vi "GetImage.vi"(0 "XRef":T4, 1 "State In":T3={"Type"=variant(bool FALSE)}) -> (14 "Image":T2, 15 "Fatal Error Out":T1)   [LabVIEW 2017, in "WriteTag.xnode"]
doc: "Write Tag XNode script that returns the picture drawn on the node."
uses:
  WriteTag.xnode
  <vilib>/XNodeSupport/XNodeXNodeRef.ctl
  State.ctl
  <vilib>/XNodeSupport/XNodeImage.ctl
  <vilib>/XNodeSupport/XNodeErrorCluster.ctl
  <vilib>/XNodeSupport/NI_XNodeSupport.lvlib
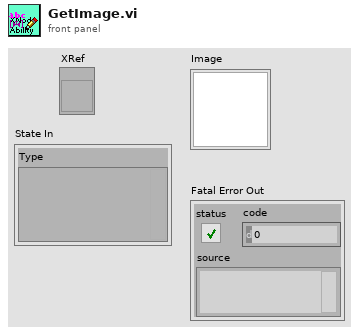
[diagram p1: front panel]
types:
  T1 = typedef "NI_XNodeSupport.lvlib/XNodeErrorCluster.ctl" = errorcluster
  T2 = typedef "NI_XNodeSupport.lvlib/XNodeImage.ctl" = picture
  T3 = typedef "WriteTag.xnode/State.ctl" = cluster{"Type":variant}
  T4 = typedef "NI_XNodeSupport.lvlib/XNodeXNodeRef.ctl" = refnum<vi>
  T5 = typedef "imagedata.ctl" = cluster{"image type":i32, "image depth":i32, "image":u8[], "mask":u8[], "colors":u32[], "Rectangle":cluster{"left":i16, "top":i16, "right":i16, "bottom":i16}}
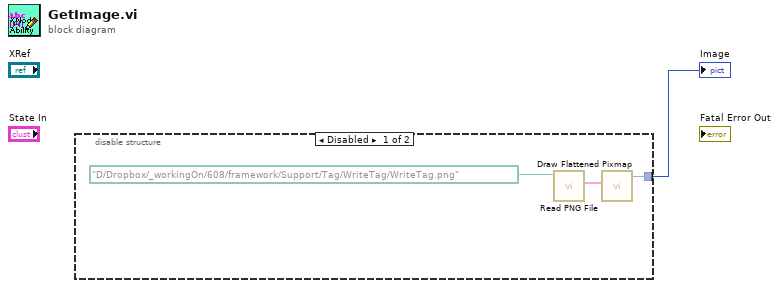
[diagram p0: block diagram]
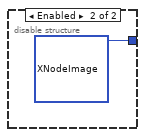
[diagram p2: hidden frame]
diagram:
  n1 = disable-structure shown="Disabled" {
    disable-tunnel: [w3 T2 bytes[3102] ("Image")] -> w1
    frame Disabled {
      n2 = call <vilib>:"Read PNG File.vi"("path to PNG file"=path "D:/Dropbox/_workingOn/608/framework/Support/Tag/WriteTag/WriteTag.png") -> ("image data"=w4:T5)  [unwired: 8 in, 2 out]
      n3 = call <vilib>:"Draw Flattened Pixmap.vi"("image data"=w4) -> ("new picture"=w3:picture)  [unwired: 8 in]
    }
    frame Enabled {
    }
  }
  "Image" <- w1
